vi "TS20171224_0845_Sub_Hall-Sensor.vi"(1 "Max_Abweichung\n(% vom richtigen Wert)":dbl=0.5 format="%#_13g", 2 "Referenzflussdichte\nB_ref_in":dbl) -> (0 "Messspannung\nU_mess_out":dbl format="%#_13g")   [LabVIEW 2018]
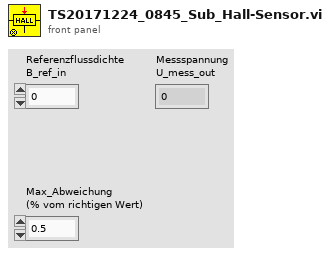
[diagram p1: front panel]
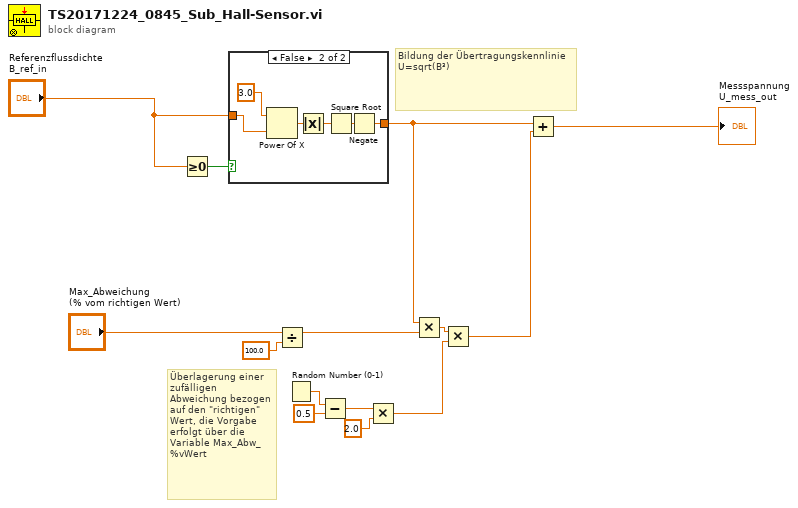
[diagram p0: block diagram]
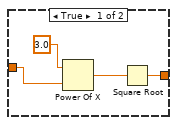
[diagram p2: hidden frame]
diagram:
  # "Bildung der Übertragungskennlinie\nU=sqrt(B³)"
  # "Überlagerung einer zufälligen Abweichung bezogen auf den \"richtigen\" Wert, die Vorgabe erfolgt über die Variable Max_Abw_%vWert"
  n1 = Greater Or Equal To 0?(x="Referenzflussdichte\nB_ref_in") -> (x >= 0?=w12:bool)
  n2 = case shown="False" w12 {
    tunnel: [w17 w19] -> w11
    tunnel: "Referenzflussdichte\nB_ref_in" -> [w16 w22]
    frame True {
      n3 = Power Of X(1:w16, 2:3.0) -> (0:w18:dbl)
      n4 = Square Root(x=w18) -> (sqrt(x)=w17:dbl)
    }
    frame False {
      n5 = Power Of X(1:w22, 2:3.0) -> (0:w24:dbl)
      n6 = Absolute Value(x=w24) -> (abs(x)=w20:dbl)
      n7 = Square Root(x=w20) -> (sqrt(x)=w23:dbl)
      n8 = Negate(x=w23) -> (-x=w19:dbl)
    }
  }
  n9 = Divide(x="Max_Abweichung\n(% vom richtigen Wert)", y=100.0) -> (x/y=w9:dbl)
  n10 = Random Number (0-1)() -> (number: 0 to 1=w1:dbl)
  n11 = Subtract(x=w1, y=0.5) -> (x-y=w6:dbl)
  n12 = Multiply(x=w6, y=2.0) -> (x*y=w8:dbl)
  n13 = Multiply(x=w11, y=w9) -> (x*y=w3:dbl)
  n14 = Multiply(x=w3, y=w8) -> (x*y=w5:dbl)
  n15 = Add(x=w11, y=w5) -> (x+y=→"Messspannung\nU_mess_out":dbl)
